vi "MV -Move indefinitely.vi"(1 "Action":bool, 8 "error in":errorcluster, 9 "Move indefinitely\nset":dbl format="%.2f", 10 "Axis #":i8=1 min=1 max=6 step=1, 11 "Address / Port":i16=1 min=1 max=31 step=1) -> (0 "error out":errorcluster, 2 "Axis out":i8=1 min=1 max=6 step=1, 3 "Address / Port out":i16=1 min=1 max=31 step=1, 4 "Query status of move\nread":string)   [LabVIEW 2014]
panel:
  # "Read"
  # "Write"
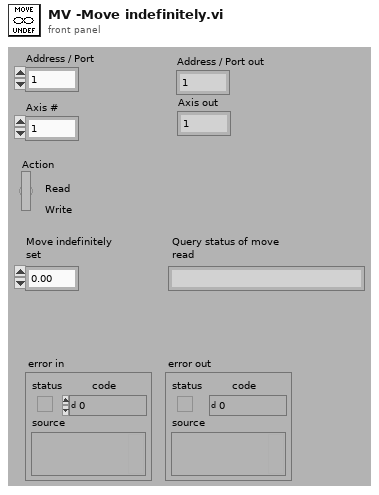
[diagram p1: front panel]
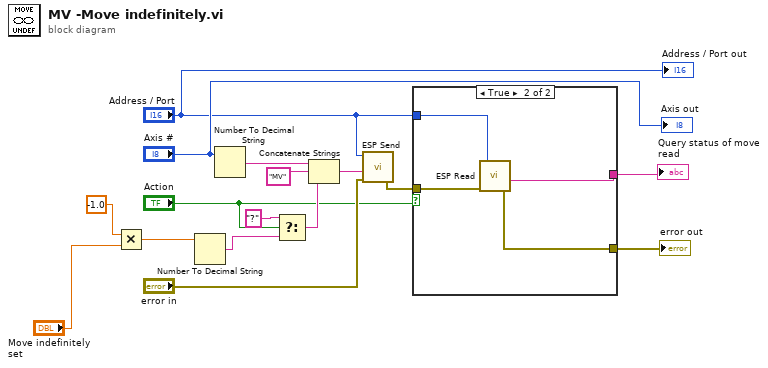
[diagram p0: block diagram]
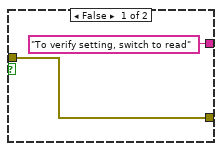
[diagram p2: hidden frame]
diagram:
  n1 = Multiply(x=-1.0, y="Move indefinitely\nset") -> (x*y=w2:dbl)
  n2 = Number To Decimal String(number=w2) -> (decimal integer string=w1:string)  [unwired: 1 in]
  n3 = Number To Decimal String(number="Axis #") -> (decimal integer string=w15:string)  [unwired: 1 in]
  n4 = Select(t="?", s="Action", f=w1) -> (s? t:f=w12:string)
  n5 = Concatenate Strings(w15, "MV" ("Substring"), w12) -> (w13:string)
  n6 = call "ESP Send.vi"("error in"="error in", "Command String"=w13, "Address / Port"="Address / Port") -> ("error out"=w7:errorcluster)  [unwired: 3 in, 1 out]
  n7 = case shown="True" "Action" {
    tunnel: "Address / Port" -> [_ w22]
    tunnel: w7 -> [w18 w21]
    tunnel: [w18 w20] -> w6
    tunnel: ["To verify setting, switch to read" w19] -> w5
    frame False {
    }
    frame True {
      n8 = call "ESP Read.vi"("error in"=w21, "Address / Port"=w22) -> ("error out"=w20:errorcluster, "Response String"=w19:string)  [unwired: 3 in, 1 out]
    }
  }
  "error out" <- w6
  "Query status of move\nread" <- w5
  "Address / Port out" <- "Address / Port"
  "Axis out" <- "Axis #"
